vi "SetTEMPCoefficients.vi"(7 "sn":string, 9 "T":dbl[](array[numeric])) -> (2 "output frame":string)   [LabVIEW 2012]
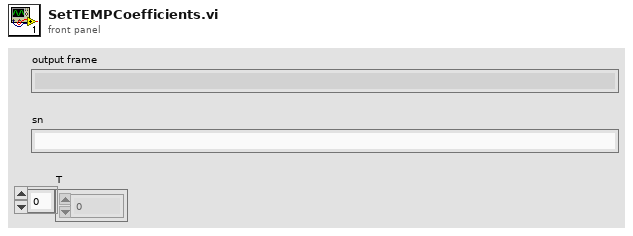
[diagram p1: front panel]
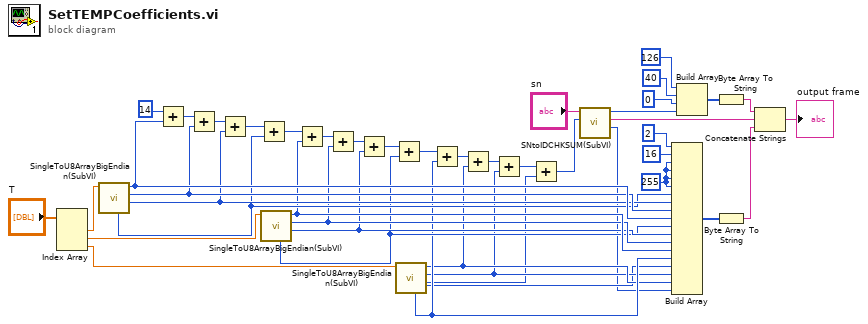
[diagram p0: block diagram]
diagram:
  w42 = u8 255
  n1 = Index Array(array="T") -> (element #1=w5:dbl, element #2=w4:dbl, element #3=w3:dbl)  [unwired: 3 in]
  n2 = call "SingleToU8ArrayBigEndian(SubVI).vi"("long data"=w5) -> ("third byte"=w25:u8, "send byte"=w28:u8, "first byte"=w29:u8, "forth byte"=w23:u8)  [unwired: 7 in]
  n3 = Add(x=u8 14, y=w29) -> (x+y=w27:u8)
  n4 = Add(x=w27, y=w28) -> (x+y=w26:u8)
  n5 = Add(x=w26, y=w25) -> (x+y=w24:u8)
  n6 = Add(x=w24, y=w23) -> (x+y=w22:u8)
  n7 = call "SingleToU8ArrayBigEndian(SubVI).vi"("long data"=w4) -> ("third byte"=w17:u8, "send byte"=w19:u8, "first byte"=w20:u8, "forth byte"=w15:u8)  [unwired: 7 in]
  n8 = Add(x=w22, y=w20) -> (x+y=w21:u8)
  n9 = Add(x=w21, y=w19) -> (x+y=w18:u8)
  n10 = Add(x=w18, y=w17) -> (x+y=w16:u8)
  n11 = Add(x=w16, y=w15) -> (x+y=w14:u8)
  n12 = call "SingleToU8ArrayBigEndian(SubVI).vi"("long data"=w3) -> ("third byte"=w7:u8, "send byte"=w8:u8, "first byte"=w9:u8, "forth byte"=w10:u8)  [unwired: 7 in]
  n13 = Add(x=w14, y=w10) -> (x+y=w13:u8)
  n14 = Add(x=w13, y=w9) -> (x+y=w12:u8)
  n15 = Add(x=w12, y=w8) -> (x+y=w11:u8)
  n16 = Add(x=w11, y=w7) -> (x+y=w2:u8)
  n17 = call "SNtoIDCHKSUM(SubVI).vi"("fix cheksum"=w2, "input sn"="sn") -> ("output check sum"=w1:u8, "output sn"=w39:string, "output id"=w36:u8)  [unwired: 7 in]
  n18 = Build Array(u8 2, u8 16, w42, w42, w42, w42, w23, w25, w28, w29, w15, w17, w19, w20, w10, w7, w8, w9, w1) -> (w43:u8[])
  n19 = Build Array(u8 126, u8 40, u8 0, w36) -> (w37:u8[])
  n20 = Byte Array To String(unsigned byte array=w37) -> (string=w38:string)
  n21 = Byte Array To String(unsigned byte array=w43) -> (string=w44:string)
  n22 = Concatenate Strings(w38, w39, w44) -> (→"output frame":string)
